vi "STEPVI - Call ATM FP Pop-up(MAIN).vi"(7 "reference":refnum<vi>, 8 "errorIn":errorcluster, 10 "file path":path, 11 "VISA":refnum<visa-resource-name>) -> (0 "errorOut":errorcluster, 2 "loginFinished？":bool, 3 "OperatorName":string)   [LabVIEW 2020]
uses:
  <vilib>/Instr/_visa.llb/VISA Configure Serial Port (Instr).vi
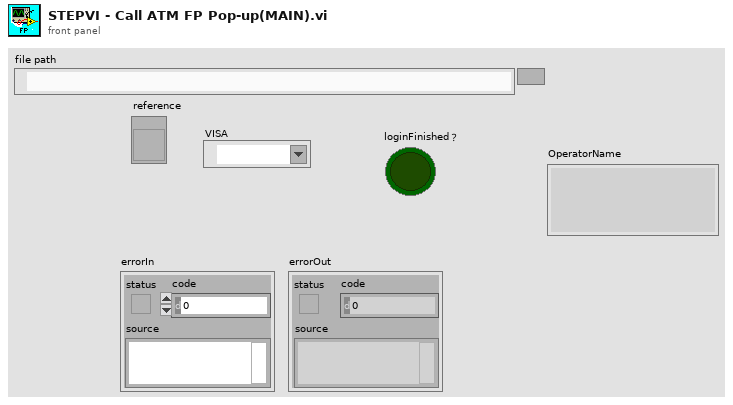
[diagram p1: front panel]
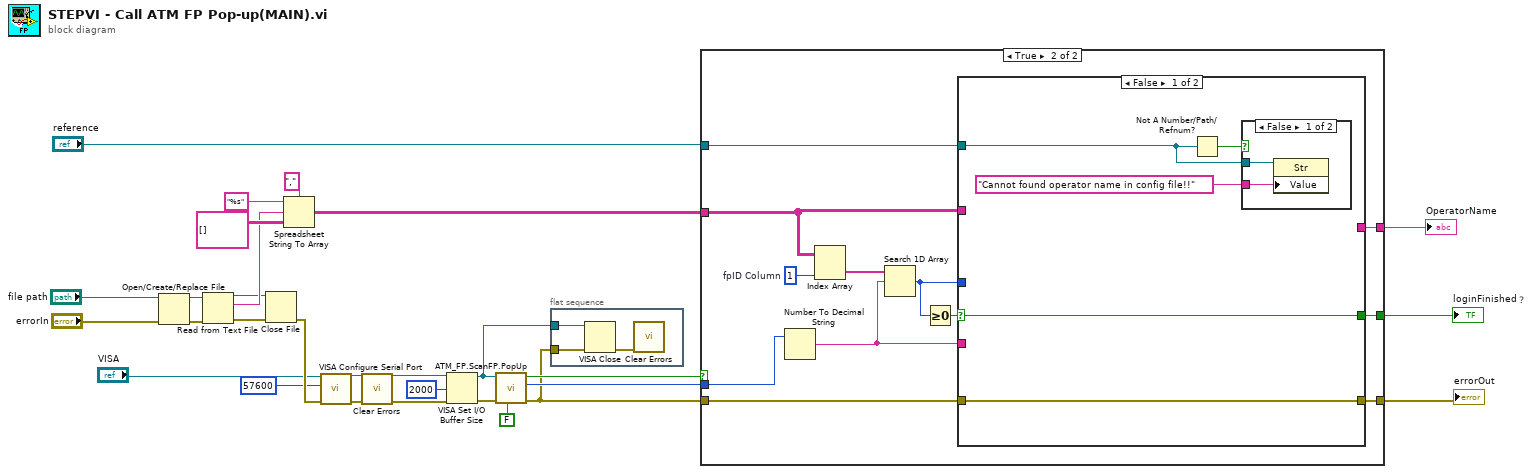
[diagram p0: block diagram]
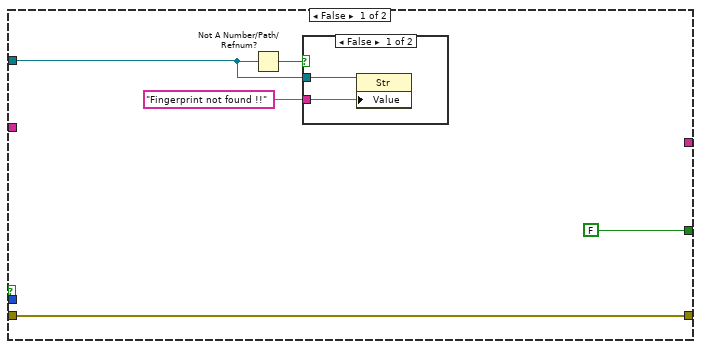
[diagram p2: hidden frame]
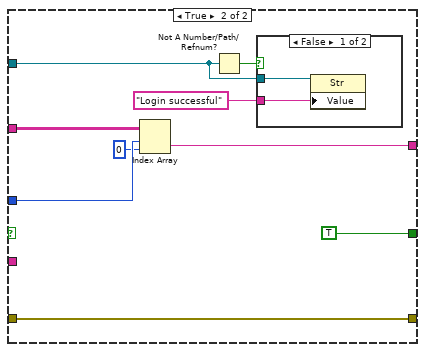
[diagram p5: hidden frame]
diagram:
  n1 = Open/Create/Replace File(file path (use dialog)="file path", error in="errorIn") -> (refnum out=w21:refnum<file>, error out=w20:errorcluster)  [unwired: 4 in, 1 out]
  n2 = Read from Text File(file (use dialog)=w21, error in=w20) -> (refnum out=w23:refnum<file>, text=w24:string, error out=w22:errorcluster)  [unwired: 2 in, 1 out]
  n3 = Close File(refnum=w23, error in=w22) -> (error out=w17:errorcluster)  [unwired: 1 out]
  n4 = Spreadsheet String To Array(delimiter (Tab)=",", format string="%s", spreadsheet string=w24, array type (2D Dbl)=string[][] []) -> (array=w19:string[][])
  n5 = call-poly "VISA Configure Serial Port"("VISA resource name"="VISA", "baud rate (9600)"=u32 57600, "error in (no error)"=w17) -> ("VISA resource name out"=w13:refnum<visa-resource-name>, "error out"=w12:errorcluster)  [unwired: 11 in]
  n6 = call <vilib>:"Clear Errors.vi"("error in (no error)"=w12) -> ("error out"=w11:errorcluster)  [unwired: 5 in, 1 out]
  n7 = VISA Set I/O Buffer Size(VISA resource name=w13, size (4096)=u32 2000 ("大小(4096)"), error in (no error)=w11) -> (VISA resource name out=w10:refnum<visa-resource-name>, error out=w16:errorcluster)  [unwired: 1 in]
  n8 = call "ATM_FP.ScanFP.PopUp.vi"("debug?"=FALSE, "errorIn"=w16, "VISA"=w10) -> ("errorOut"=w9:errorcluster, "fpID"=w28:u16, "fpFound"=w18:bool)  [unwired: 6 in]
  n9 = flat-sequence {
    tunnel: w10 -> [w31]
    tunnel: w9 -> [w29]
    frame #0 {
      n10 = VISA Close(VISA resource name=w31, error in (no error)=w29) -> (error out=w30:errorcluster)
      n11 = call <vilib>:"Clear Errors.vi"("error in (no error)"=w30) -> ()  [unwired: 5 in, 2 out]
    }
  }
  n12 = case shown="True" w18 {
    tunnel: "reference" -> [w34 w45]
    tunnel: [_ w44] -> w4
    tunnel: [FALSE w43] -> w3
    tunnel: w28 -> [_ w42]
    tunnel: w19 -> [_ w41]
    tunnel: w9 -> [w32 w40]
    tunnel: [w32 w39] -> w5
    frame False {
      n13 = Not A Number/Path/Refnum?(number/path/refnum=w34) -> (NaN/Path/Refnum?=w35:bool)
      n14 = case shown="False" w35 {
        tunnel: "Fingerprint not found !!" ("Value") -> [w38 _]
        tunnel: w34 -> [w37 _]
        frame False {
          n15 = property class="Str"(reference=w37, "Value"=w38) -> ()  [unwired: 1 in, 2 out]
        }
        frame True {
        }
      }
    }
    frame True {
      w50 = 1  # fpID Column
      n16 = Number To Decimal String(number=w42) -> (decimal integer string=w46:string)  [unwired: 1 in]
      n17 = Index Array(array=w41, index (col)=w50) -> (element=w49:string[])  [unwired: 1 in]
      n18 = Search 1D Array(1D array=w49, element=w46) -> (index of element=w47:i32)  [unwired: 1 in]
      n19 = Greater Or Equal To 0?(x=w47) -> (x >= 0?=w48:bool)
      n20 = case shown="False" w48 {
        selector: w48 -> [w52 _]
        tunnel: w41 -> [_ w66]
        tunnel: w47 -> [_ w65]
        tunnel: w46 -> [_ _]
        tunnel: w45 -> [w53 w62]
        tunnel: [_ w60] -> w44
        tunnel: [w52 TRUE] -> w43
        tunnel: w40 -> [w51 w59]
        tunnel: [w51 w59] -> w39
        frame False {
          n21 = Not A Number/Path/Refnum?(number/path/refnum=w53) -> (NaN/Path/Refnum?=w54:bool)
          n22 = case shown="False" w54 {
            tunnel: "Cannot found operator name in config file!!" ("Value") -> [w57 _]
            tunnel: w53 -> [w56 _]
            frame False {
              n23 = property class="Str"(reference=w56, "Value"=w57) -> ()  [unwired: 1 in, 2 out]
            }
            frame True {
            }
          }
        }
        frame True {
          n24 = Index Array(array=w66, index (row)=w65, index (col)=0 ("disabled index (col)")) -> (element=w60:string)
          n25 = Not A Number/Path/Refnum?(number/path/refnum=w62) -> (NaN/Path/Refnum?=w63:bool)
          n26 = case shown="False" w63 {
            tunnel: "Login successful" ("Value") -> [w68 _]
            tunnel: w62 -> [w67 _]
            frame False {
              n27 = property class="Str"(reference=w67, "Value"=w68) -> ()  [unwired: 1 in, 2 out]
            }
            frame True {
            }
          }
        }
      }
    }
  }
  "errorOut" <- w5
  "OperatorName" <- w4
  "loginFinished？" <- w3
